vi "WriteTempData.vi"(2 "rawdata":T1, 3 "Enum":enum16{"create new", "write", "close"}(ring), 6 "error in (no error)":errorcluster) -> (1 "offset":i32, 5 "error out":errorcluster)   [LabVIEW 2009]
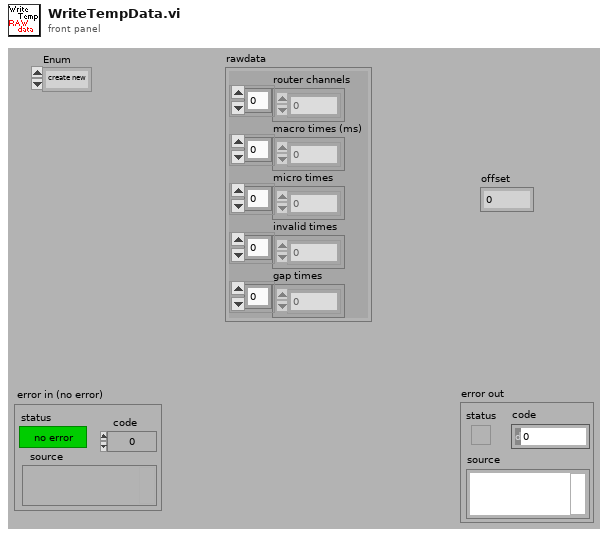
[diagram p1: front panel]
types:
  T1 = cluster{"router channels":u8[], "macro times (ms)":dbl[], "micro times":u16[], "invalid times":dbl[], "gap times":dbl[]}
  T2 = cluster{"router":u8[], "macro times":dbl[], "micro times":u16[], "invalid":dbl[], "gap":dbl[]}
  T3 = enum16{"open", "replace", "create", "open or create", "replace or create", "replace or create with confirmation"}
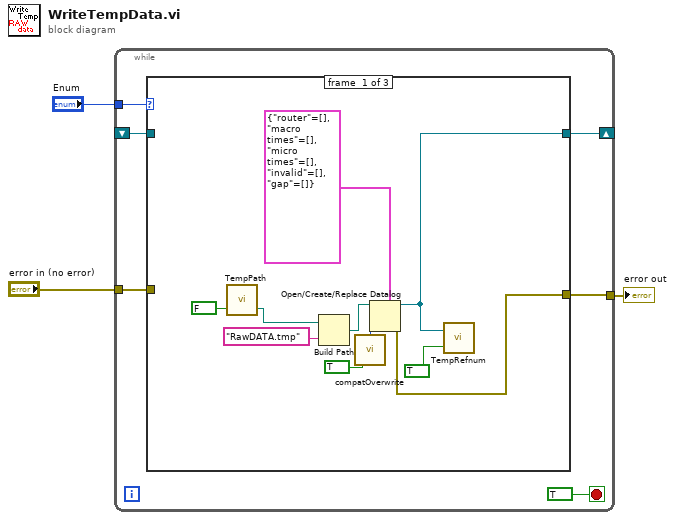
[diagram p0: block diagram]
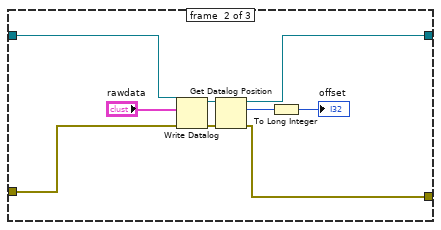
[diagram p2: hidden frame]
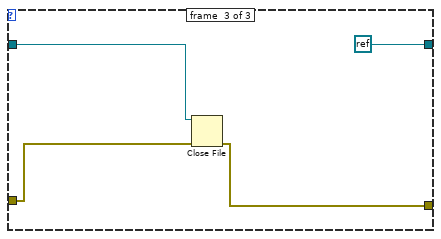
[diagram p3: hidden frame]
diagram:
  n1 = while {
    tunnel: "Enum" -> [w9]
    tunnel: [w7] -> w2
    tunnel: "error in (no error)" -> [w6]
    shift-right: [w5] -> _
    shift-left: _ -> [w4]
    stop <- TRUE stop-if-true
    n2 = case shown="\"write\", Default" w9 {
      tunnel: [w12 w25 w31] -> w7
      tunnel: w6 -> [_ w26 w32]
      tunnel: [w11 w23 refnum<k0> refnum] -> w5
      tunnel: w4 -> [_ w24 w30]
      frame #0 {
        n3 = call "TempPath.vi"("change"=FALSE) -> ("stripped path 2"=w15:path)  [unwired: 2 in]
        n4 = Build Path(base path=w15, name or relative path="RawDATA.tmp" ("prompt")) -> (appended path=w17:path)
        n5 = call <vilib>:"compatOverwrite.vi"("overwrite (F)"=TRUE) -> ("overwrite?"=w10:T3)
        n6 = Open/Create/Replace Datalog(5:T2 {"router"=[], "macro times"=[], "micro times"=[], "invalid"=[], "gap"=[]} ("cluster"), 10:w10, 11:w17) -> (0:w12:errorcluster, 3:w11:refnum<k1>)  [unwired: 3 in, 1 out]
        n7 = call "TempRefnum.vi"("change?"=TRUE, "refnum in"=w11) -> ()  [unwired: 1 out]
      }
      frame #1 {
        n8 = Write Datalog(4:w26, 6:"rawdata", 7:w24) -> (0:w21:errorcluster, 3:w22:refnum<k1>)
        n9 = Get Datalog Position(4:w21, 7:w22) -> (0:w25:errorcluster, 2:w20:i64, 3:w23:refnum<k1>)
        n10 = To Long Integer(number=w20) -> (32bit integer=→"offset":i32)
      }
      frame #2 {
        n11 = Close File(refnum=w30, error in=w32) -> (error out=w31:errorcluster)  [unwired: 1 out]
      }
    }
  }
  "error out" <- w2
